vi "Read Read Only.vi"(8 "error in (no error)":errorcluster, 11 "Abs_Value in":refnum<class "Abs_Value_1D.lvclass">) -> (0 "error out":errorcluster, 2 "Read Only":bool, 3 "Abs_Value out":refnum<class "Abs_Value_1D.lvclass">)   [LabVIEW 2021, in "Abs_Value_1D.lvclass"]
uses:
  Abs_Value_1D.lvclass
  Abs_Value_1D.lvclass/Abs_Value_1D.ctl
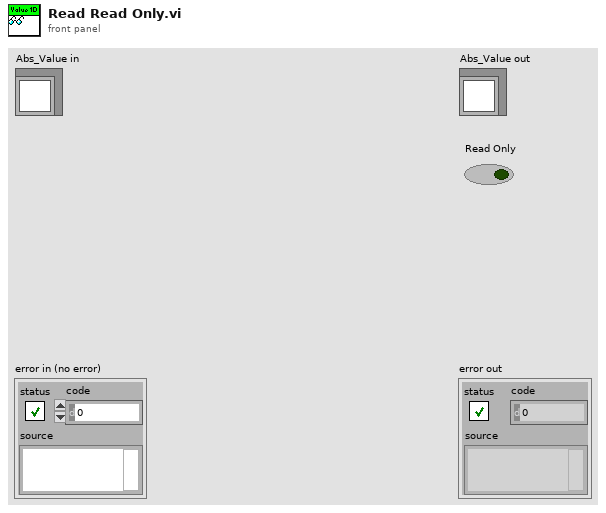
[diagram p1: front panel]
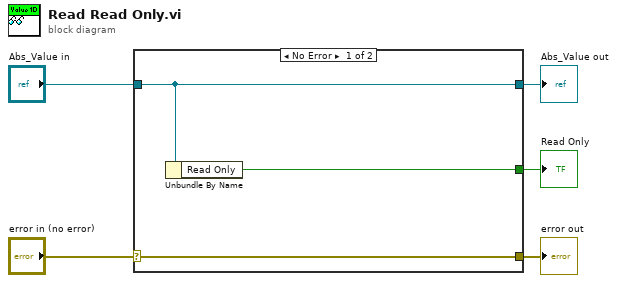
[diagram p0: block diagram]
diagram:
  n1 = case shown="No Error" "error in (no error)" {
    selector: "error in (no error)" -> [w8 w9]
    tunnel: [w8 w9] -> w4
    tunnel: [w7 w10] -> w2
    tunnel: "Abs_Value in" -> [w7 w10]
    tunnel: [w6 _] -> w1
    frame No Error {
      n2 = Unbundle By Name(w7) -> ("Read Only"=w6:bool)
    }
    frame Error {
    }
  }
  "error out" <- w4
  "Abs_Value out" <- w2
  "Read Only" <- w1
